vi "Byte Buffer.Read.Typed Array.vi"(0 "Byte Buffer in":refnum<class "Byte Buffer.lvclass">, 1 "data type":T1, 5 "buffer in":dbl[](array[numeric]), 7 "count":i32, 9 "buffer offset":u64, 11 "error in (no error)":errorcluster) -> (4 "Byte Buffer out":refnum<class "Byte Buffer.lvclass">, 6 "buffer out":dbl[](array[numeric]), 10 "new buffer offset":u64, 15 "error out":errorcluster)   [LabVIEW 2016, in "VeriStand Data.lvlib" / "Byte Buffer.lvclass"]
uses:
  Byte Buffer.lvclass
  Typedefs/Typedefs.Data Types.ctl
  Byte Buffer.lvclass/Byte Buffer.ctl
  Byte Buffer.Read (1D Boolean).vi
  Type Conversion/Type Conversion.To Double.Subset (1D Boolean).vi
  Byte Buffer.Read (1D SGL).vi
  Type Conversion/Type Conversion.To Double.Subset (1D SGL).vi
  Byte Buffer.Read (1D DBL).vi
  Byte Buffer.Read (1D I8).vi
  Type Conversion/Type Conversion.To Double.Subset (1D I8).vi
  Byte Buffer.Read (1D I16).vi
  Type Conversion/Type Conversion.To Double.Subset (1D I16).vi
  Byte Buffer.Read (1D I32).vi
  Type Conversion/Type Conversion.To Double.Subset (1D I32).vi
  Byte Buffer.Read (1D I64).vi
  Type Conversion/Type Conversion.To Double.Subset (1D I64).vi
  Byte Buffer.Read (1D U8).vi
  Type Conversion/Type Conversion.To Double.Subset (1D U8).vi
  Byte Buffer.Read (1D U16).vi
  Type Conversion/Type Conversion.To Double.Subset (1D U16).vi
  Byte Buffer.Read (1D U32).vi
  Type Conversion/Type Conversion.To Double.Subset (1D U32).vi
  Byte Buffer.Read (1D U64).vi
  Type Conversion/Type Conversion.To Double.Subset (1D U64).vi
  Utilities/Utilities.Sizeof.Scalar.vi
  Byte Buffer.Read (String).vi
  Type Conversion/Type Conversion.To Double.vi
  Type Conversion/Type Conversion.To Double (1D Boolean).vi
  Type Conversion/Type Conversion.To Double (1D SGL).vi
  Type Conversion/Type Conversion.To Double (1D I8).vi
  Type Conversion/Type Conversion.To Double (1D I16).vi
  Type Conversion/Type Conversion.To Double (1D I32).vi
  Type Conversion/Type Conversion.To Double (1D I64).vi
  Type Conversion/Type Conversion.To Double (1D U8).vi
  Type Conversion/Type Conversion.To Double (1D U16).vi
  Type Conversion/Type Conversion.To Double (1D U32).vi
  Type Conversion/Type Conversion.To Double (1D U64).vi
  Byte Buffer.Allocate.vi
  Byte Buffer.Get Buffer Subset.vi
  Memory Management/Memory Management.MoveByteBlock.Write (String).vi
  Memory Management/Memory Management.Handle Return.vi
  VeriStand Data.lvlib
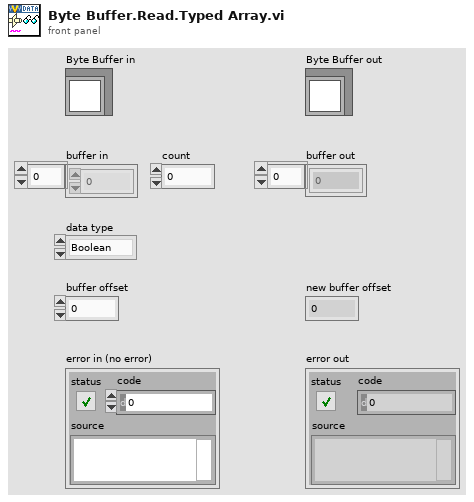
[diagram p1: front panel]
types:
  T1 = typedef "VeriStand Data.lvlib/Typedefs.Data Types.ctl" = enum16{"Boolean", "Single", "Double", "I8", "I16", "I32", "I64", "U8", "U16", "U32", "U64"}
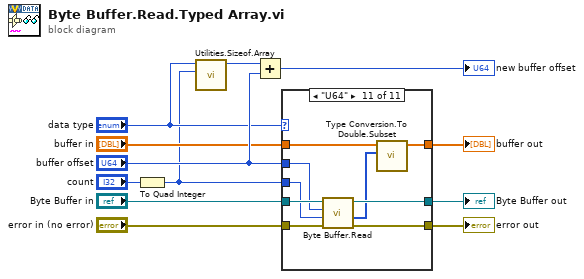
[diagram p0: block diagram]
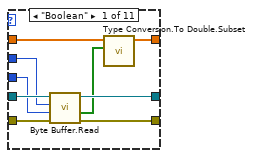
[diagram p2: hidden frame]
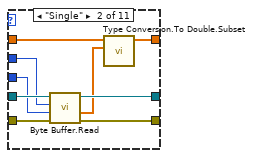
[diagram p3: hidden frame]
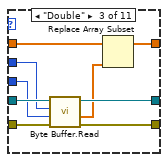
[diagram p4: hidden frame]
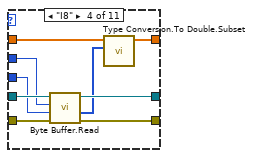
[diagram p5: hidden frame]
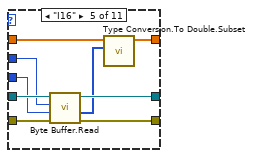
[diagram p6: hidden frame]
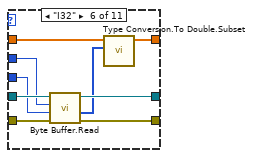
[diagram p7: hidden frame]
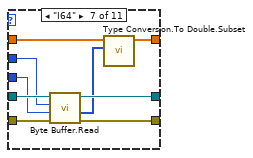
[diagram p8: hidden frame]
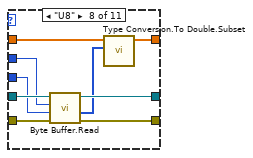
[diagram p9: hidden frame]
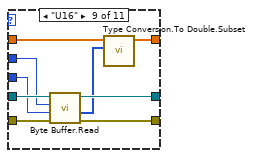
[diagram p10: hidden frame]
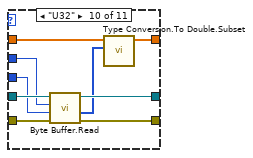
[diagram p11: hidden frame]
diagram:
  n1 = To Quad Integer(1:"count") -> (0:w1:i64)
  n2 = call "Utilities.Sizeof.Array.vi"("count"=w1, "data type"="data type") -> ("size"=w5:u64)  [unwired: 9 in]
  n3 = Add(x=w5, y="buffer offset") -> (x+y=→"new buffer offset":u64)
  n4 = case shown="\"U64\"" "data type" {
    tunnel: "buffer offset" -> [w20 w29 w38 w47 w56 w65 w74 w83 w92 w101 w110]
    tunnel: "Byte Buffer in" -> [w21 w30 w39 w48 w57 w66 w75 w84 w93 w102 w111]
    tunnel: [w14 w23 w34 w41 w50 w59 w68 w77 w86 w95 w104] -> w11
    tunnel: "error in (no error)" -> [w19 w28 w37 w46 w55 w64 w73 w82 w91 w100 w109]
    tunnel: [w17 w26 w35 w44 w53 w62 w71 w80 w89 w98 w107] -> w9
    tunnel: w1 -> [w18 w27 w36 w45 w54 w63 w72 w81 w90 w99 w108]
    tunnel: [w16 w25 w32 w43 w52 w61 w70 w79 w88 w97 w106] -> w7
    tunnel: "buffer in" -> [w15 w24 w33 w42 w51 w60 w69 w78 w87 w96 w105]
    frame "Boolean" {
      n5 = call-poly "Byte Buffer.Read.vi"("error in (no error)"=w19, "count"=w18, "buffer offset"=w20, "Byte Buffer in"=w21) -> ("error out"=w17:errorcluster, "value"=w13:bool[], "Byte Buffer out"=w14:refnum<class "Byte Buffer.lvclass">)  [unwired: 5 in]
      n6 = call-poly "Type Conversion.To Double.Subset.vi"("new values"=w13, "values in"=w15) -> ("values out"=w16:dbl[])  [unwired: 9 in]
    }
    frame "Single" {
      n7 = call-poly "Byte Buffer.Read.vi"("error in (no error)"=w28, "count"=w27, "buffer offset"=w29, "Byte Buffer in"=w30) -> ("error out"=w26:errorcluster, "value"=w22:sgl[], "Byte Buffer out"=w23:refnum<class "Byte Buffer.lvclass">)  [unwired: 5 in]
      n8 = call-poly "Type Conversion.To Double.Subset.vi"("new values"=w22, "values in"=w24) -> ("values out"=w25:dbl[])  [unwired: 9 in]
    }
    frame "Double" {
      n9 = call-poly "Byte Buffer.Read.vi"("error in (no error)"=w37, "count"=w36, "buffer offset"=w38, "Byte Buffer in"=w39) -> ("error out"=w35:errorcluster, "value"=w31:dbl[], "Byte Buffer out"=w34:refnum<class "Byte Buffer.lvclass">)  [unwired: 5 in]
      n10 = Replace Array Subset(array=w33, new element=w31) -> (w32:dbl[])  [unwired: 1 in]
    }
    frame "I8" {
      n11 = call-poly "Byte Buffer.Read.vi"("error in (no error)"=w46, "count"=w45, "buffer offset"=w47, "Byte Buffer in"=w48) -> ("error out"=w44:errorcluster, "value"=w40:i8[], "Byte Buffer out"=w41:refnum<class "Byte Buffer.lvclass">)  [unwired: 5 in]
      n12 = call-poly "Type Conversion.To Double.Subset.vi"("new values"=w40, "values in"=w42) -> ("values out"=w43:dbl[])  [unwired: 9 in]
    }
    frame "I16" {
      n13 = call-poly "Byte Buffer.Read.vi"("error in (no error)"=w55, "count"=w54, "buffer offset"=w56, "Byte Buffer in"=w57) -> ("error out"=w53:errorcluster, "value"=w49:i16[], "Byte Buffer out"=w50:refnum<class "Byte Buffer.lvclass">)  [unwired: 5 in]
      n14 = call-poly "Type Conversion.To Double.Subset.vi"("new values"=w49, "values in"=w51) -> ("values out"=w52:dbl[])  [unwired: 9 in]
    }
    frame "I32" {
      n15 = call-poly "Byte Buffer.Read.vi"("error in (no error)"=w64, "count"=w63, "buffer offset"=w65, "Byte Buffer in"=w66) -> ("error out"=w62:errorcluster, "value"=w58:i32[], "Byte Buffer out"=w59:refnum<class "Byte Buffer.lvclass">)  [unwired: 5 in]
      n16 = call-poly "Type Conversion.To Double.Subset.vi"("new values"=w58, "values in"=w60) -> ("values out"=w61:dbl[])  [unwired: 9 in]
    }
    frame "I64" {
      n17 = call-poly "Byte Buffer.Read.vi"("error in (no error)"=w73, "count"=w72, "buffer offset"=w74, "Byte Buffer in"=w75) -> ("error out"=w71:errorcluster, "value"=w67:i64[], "Byte Buffer out"=w68:refnum<class "Byte Buffer.lvclass">)  [unwired: 5 in]
      n18 = call-poly "Type Conversion.To Double.Subset.vi"("new values"=w67, "values in"=w69) -> ("values out"=w70:dbl[])  [unwired: 9 in]
    }
    frame "U8" {
      n19 = call-poly "Byte Buffer.Read.vi"("error in (no error)"=w82, "count"=w81, "buffer offset"=w83, "Byte Buffer in"=w84) -> ("error out"=w80:errorcluster, "value"=w76:u8[], "Byte Buffer out"=w77:refnum<class "Byte Buffer.lvclass">)  [unwired: 5 in]
      n20 = call-poly "Type Conversion.To Double.Subset.vi"("new values"=w76, "values in"=w78) -> ("values out"=w79:dbl[])  [unwired: 9 in]
    }
    frame "U16" {
      n21 = call-poly "Byte Buffer.Read.vi"("error in (no error)"=w91, "count"=w90, "buffer offset"=w92, "Byte Buffer in"=w93) -> ("error out"=w89:errorcluster, "value"=w85:u16[], "Byte Buffer out"=w86:refnum<class "Byte Buffer.lvclass">)  [unwired: 5 in]
      n22 = call-poly "Type Conversion.To Double.Subset.vi"("new values"=w85, "values in"=w87) -> ("values out"=w88:dbl[])  [unwired: 9 in]
    }
    frame "U32" {
      n23 = call-poly "Byte Buffer.Read.vi"("error in (no error)"=w100, "count"=w99, "buffer offset"=w101, "Byte Buffer in"=w102) -> ("error out"=w98:errorcluster, "value"=w94:u32[], "Byte Buffer out"=w95:refnum<class "Byte Buffer.lvclass">)  [unwired: 5 in]
      n24 = call-poly "Type Conversion.To Double.Subset.vi"("new values"=w94, "values in"=w96) -> ("values out"=w97:dbl[])  [unwired: 9 in]
    }
    frame "U64" {
      n25 = call-poly "Byte Buffer.Read.vi"("error in (no error)"=w109, "count"=w108, "buffer offset"=w110, "Byte Buffer in"=w111) -> ("error out"=w107:errorcluster, "value"=w103:u64[], "Byte Buffer out"=w104:refnum<class "Byte Buffer.lvclass">)  [unwired: 5 in]
      n26 = call-poly "Type Conversion.To Double.Subset.vi"("new values"=w103, "values in"=w105) -> ("values out"=w106:dbl[])  [unwired: 9 in]
    }
  }
  "error out" <- w9
  "Byte Buffer out" <- w11
  "buffer out" <- w7
